vi "Drive Axis Modifications.vi"(1 "Driver JoyStick Info":T2) -> (0 "Driver JoyStick Info 2":T2)   [LabVIEW 2012]
uses:
  <vilib>/Rock Robotics/WPI/Solenoid/WPI_SolenoidValue.ctl
  Drive Global Data.vi
panel:
  # "X"
  # "Y"
  # "X"
  # "Y"
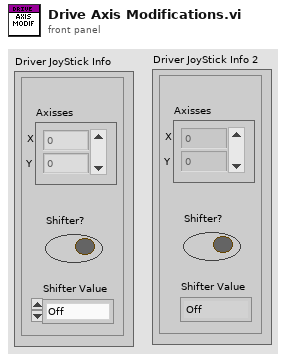
[diagram p1: front panel]
types:
  T1 = typedef "WPI_SolenoidValue.ctl" = enum16{"Off", "On", "Forward", "Reverse"}
  T2 = cluster{"Shifter?":bool, "Axisses":dbl[], "Shifter Value":T1}
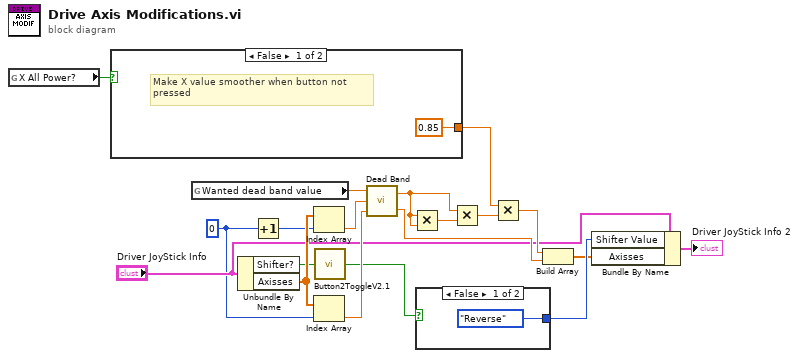
[diagram p0: block diagram]
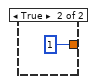
[diagram p2: hidden frame]
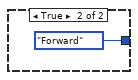
[diagram p3: hidden frame]
diagram:
  w2 = 0 ("index")
  n1 = global read "Drive Global Data.vi" "X All Power?"() -> (w12:bool)
  n2 = case shown="False" w12 {
    tunnel: [0.85 1] -> w13
    frame False {
      # "Make X value smoother when button not \npressed"
    }
    frame True {
    }
  }
  n3 = global read "Drive Global Data.vi" "Wanted dead band value"() -> (w16:dbl)
  n4 = Unbundle By Name("Driver JoyStick Info") -> ("Shifter?"=w4:bool, "Axisses"=w19:dbl[])
  n5 = Increment(x=w2) -> (x+1=w1:i32)
  n6 = Index Array(array=w19, index=w1) -> (element=w15:dbl)
  n7 = Index Array(array=w19, index=w2) -> (element=w14:dbl)
  n8 = call "Button2ToggleV2.1.vi"("a"=w4) -> ("Result(clone)"=w3:bool)
  n9 = call "Dead Band.vi"("Axis 2 In"=w14, "Axis 1 In"=w15, "Dead Band"=w16) -> ("Axis 2 Out"=w17:dbl, "Axis 1 Out"=w10:dbl)
  n10 = Multiply(x=w10, y=w10) -> (x*y=w11:dbl)
  n11 = case shown="False" w3 {
    tunnel: [WPI_SolenoidValue."Reverse" ("Value") WPI_SolenoidValue."Forward" ("Value")] -> w6
    frame False {
    }
    frame True {
    }
  }
  n12 = Multiply(x=w10, y=w11) -> (x*y=w9:dbl)
  n13 = Multiply(x=w13, y=w9) -> (x*y=w18:dbl)
  n14 = Build Array(w18, w17) -> (w5:dbl[])
  n15 = Bundle By Name(cluster="Driver JoyStick Info", "Shifter Value"=w6, "Axisses"=w5) -> (→"Driver JoyStick Info 2":T2)
